vi "Instruction-SupportStateData.vi"(0 "ERP-CreateInstructions in":refnum<class "ERP-CreateInstructions.lvclass">, 6 "Manufacturing Tree - Instruction Sets":refnum<vi>, 8 "Inspection Tree - Instruction Sets":refnum<vi>, 10 "General Tree - Instruction Sets":refnum<vi>) -> (14 "ERP-CreateInstructions out":refnum<class "ERP-CreateInstructions.lvclass">)   [LabVIEW 2013, in "ERP-CreateInstructions.lvclass"]
uses:
  ERP-CreateInstructions.lvclass
  ERP-CreateInstructions.lvclass/ERP-CreateInstructions.ctl
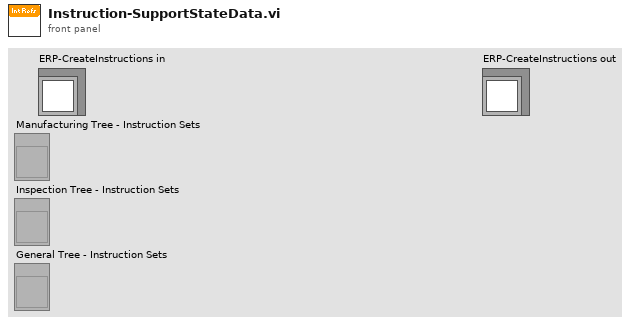
[diagram p1: front panel]
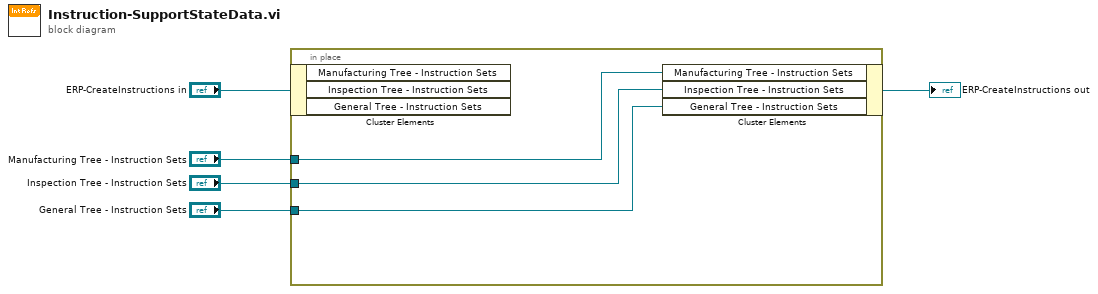
[diagram p0: block diagram]
diagram:
  n1 = in-place {
    in-place-border: "Manufacturing Tree - Instruction Sets" -> [w8]
    in-place-border: "Inspection Tree - Instruction Sets" -> [w7]
    in-place-border: "General Tree - Instruction Sets" -> [w6]
    n2 = in-place-cluster #1("ERP-CreateInstructions in") -> ()  [unwired: 3 out]
    n3 = in-place-cluster #1("Manufacturing Tree - Instruction Sets"=w8, "Inspection Tree - Instruction Sets"=w7, "General Tree - Instruction Sets"=w6) -> (→"ERP-CreateInstructions out":refnum<class "ERP-CreateInstructions.lvclass">)
  }
